vi "Configure Arbitrary Waveform.vi"(7 "Waveform Shape (0: Square)":i32(ring) items=["Square"], 8 "error in (no error)":errorcluster, 9 "Waveform Number (1)":i32=1, 10 "Channel (1: Channel 1)":i32(ring)=1 items=["Channel 1"=1, "Channel 2"=2], 11 "VISA resource name":refnum<visa-resource-name>) -> (0 "error out":errorcluster, 3 "VISA resource name out":refnum<visa-resource-name>)   [LabVIEW 2012, in "Keysight B2980 Series.lvlib"]
doc: "Configure the arbitrary waveform output.\n\n<b>Note(s):</b>\nThis VI is only applicable for model B2985A and B2987A."
uses:
  Keysight B2980 Series.lvlib
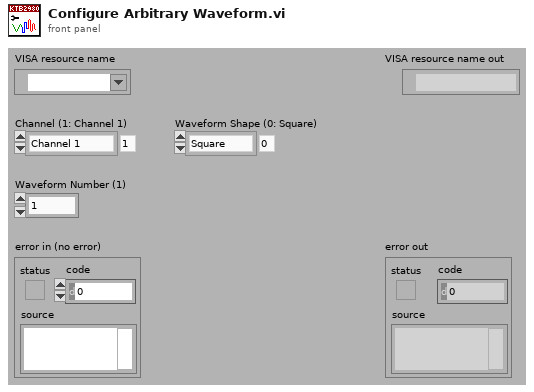
[diagram p1: front panel]
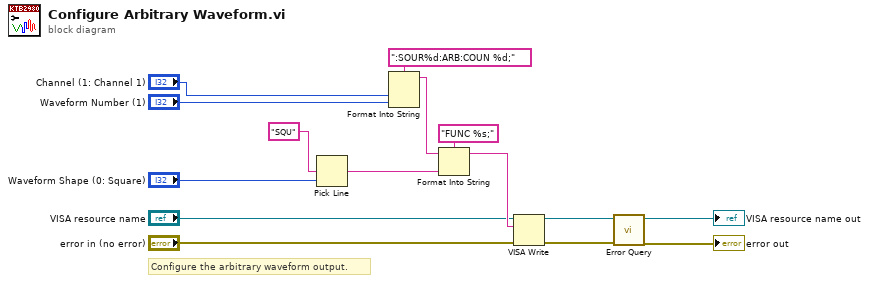
[diagram p0: block diagram]
diagram:
  # "Configure the arbitrary waveform output."
  n1 = Pick Line(multi-line string="SQU", line index="Waveform Shape (0: Square)") -> (output string=w3:string)  [unwired: 1 out]
  n2 = Format Into String(format string=":SOUR%d:ARB:COUN %d;", "Channel (1: Channel 1)", "Waveform Number (1)") -> (resulting string=w12:string)  [unwired: 2 in, 1 out]
  n3 = Format Into String(format string="FUNC %s;", initial string=w12, w3) -> (resulting string=w10:string)  [unwired: 1 in, 1 out]
  n4 = VISA Write(VISA resource name="VISA resource name", write buffer=w10, error in (no error)="error in (no error)") -> (VISA resource name out=w7:refnum<visa-resource-name>, error out=w6:errorcluster)  [unwired: 1 out]
  n5 = call "Error Query.vi"("error in (no error)"=w6, "VISA resource name"=w7) -> ("error out"=→"error out":errorcluster, "VISA resource name out"=→"VISA resource name out":refnum<visa-resource-name>)  [unwired: 8 out]
